vi "DAQ_pp3c_AudioLoadBuffersTasks.vi"(5 "Daq status in":T1={"Sound AO"="Dev6/ao0", "Shock intesity AO"="Dev6/ao1", "Code_LED DO"="Dev6/port1:2", "Switch DI"="Dev6/port1/line0", "Webcam"="cam9", "Sound AO task"="", "Sound card task"=0, "Shock intensity AO task"="", "Code_LED DO task"="", "Switch DI task"="", "AO <=> Sound card"=FALSE, "Sound card"=0, "sample rate"=100000.0, "Variable shock"=TRUE, "Webcam on"=FALSE, "Waveform memo"={"t0"=timestamp(0 s since 1904-01-01), "dt"=1.0, "Y"=[]}, "Tone trigger"="PFI1", "Master-9 DO"="PFI1", "Master-9 DO task"="Dev6/port0/line5:7", "Master-9 on"=TRUE} {"sample rate" min=8000.0; "Sound card task" format="%.0x"}, 7 "Waveform":waveform(dbl), 11 "error in (no error)":errorcluster) -> (6 "Daq status out":T1={"Sound AO"="Dev6/ao0", "Shock intesity AO"="Dev6/ao1", "Code_LED DO"="Dev6/port1:2", "Switch DI"="Dev6/port1/line0", "Webcam"="cam9", "Sound AO task"="", "Sound card task"=0, "Shock intensity AO task"="", "Code_LED DO task"="", "Switch DI task"="", "AO <=> Sound card"=FALSE, "Sound card"=0, "sample rate"=100000.0, "Variable shock"=TRUE, "Webcam on"=FALSE, "Waveform memo"={"t0"=timestamp(0 s since 1904-01-01), "dt"=1.0, "Y"=[]}, "Tone trigger"="PFI1", "Master-9 DO"="PFI1", "Master-9 DO task"="Dev6/port0/line5:7", "Master-9 on"=TRUE} {"sample rate" min=8000.0; "Sound card task" format="%.0x"}, 15 "error out":errorcluster)   [LabVIEW 2013]
uses:
  CTL_pp3c_DaqStatus.ctl
  <vilib>/userdefined/High Color/IMAQdx.ctl
  <vilib>/sound2/lvsound2.llb/Sound Output Task ID.ctl
  <vilib>/DAQmx/write.llb/DAQmx Write (Analog Wfm 1Chan NSamp).vi
  <vilib>/DAQmx/create/channels.llb/DAQmx Create Channel (AO-Voltage-Basic).vi
  <vilib>/DAQmx/configure/timing.llb/DAQmx Timing (Use Waveform).vi
  <vilib>/DAQmx/miscellaneous.llb/DAQmx Fill In Error Info.vi
  <resource>/objmgr/daqmx.rc
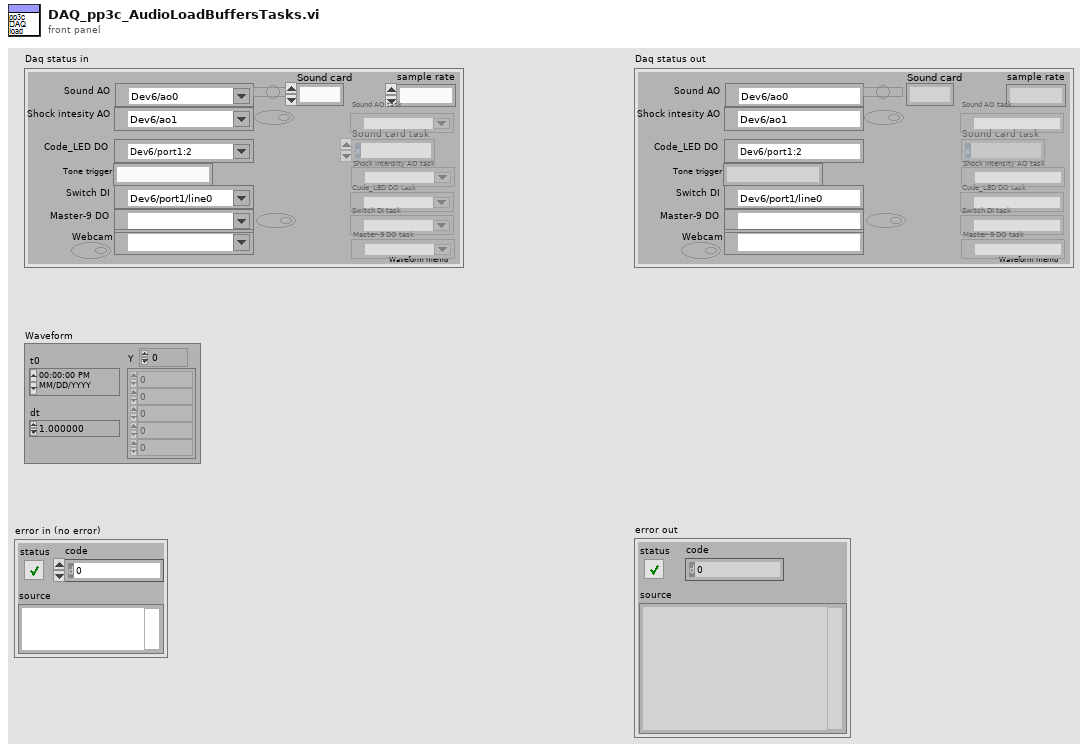
[diagram p1: front panel]
types:
  T1 = typedef "CTL_pp3c_DaqStatus.ctl" = cluster{"Sound AO":tag, "Shock intesity AO":tag, "Code_LED DO":tag, "Switch DI":tag, "Webcam":T2, "Sound AO task":refnum<k21>, "Sound card task":T3, "Shock intensity AO task":refnum<k21>, "Code_LED DO task":refnum<k21>, "Switch DI task":refnum<k21>, "AO <=> Sound card":bool, "Sound card":u32, "sample rate":dbl, "Variable shock":bool, "Webcam on":bool, "Waveform memo":waveform(dbl), "Tone trigger":string, "Master-9 DO":tag, "Master-9 DO task":refnum<k21>, "Master-9 on":bool}
  T2 = typedef "IMAQdx.ctl" = refnum<k21>
  T3 = typedef "Sound Output Task ID.ctl" = u32
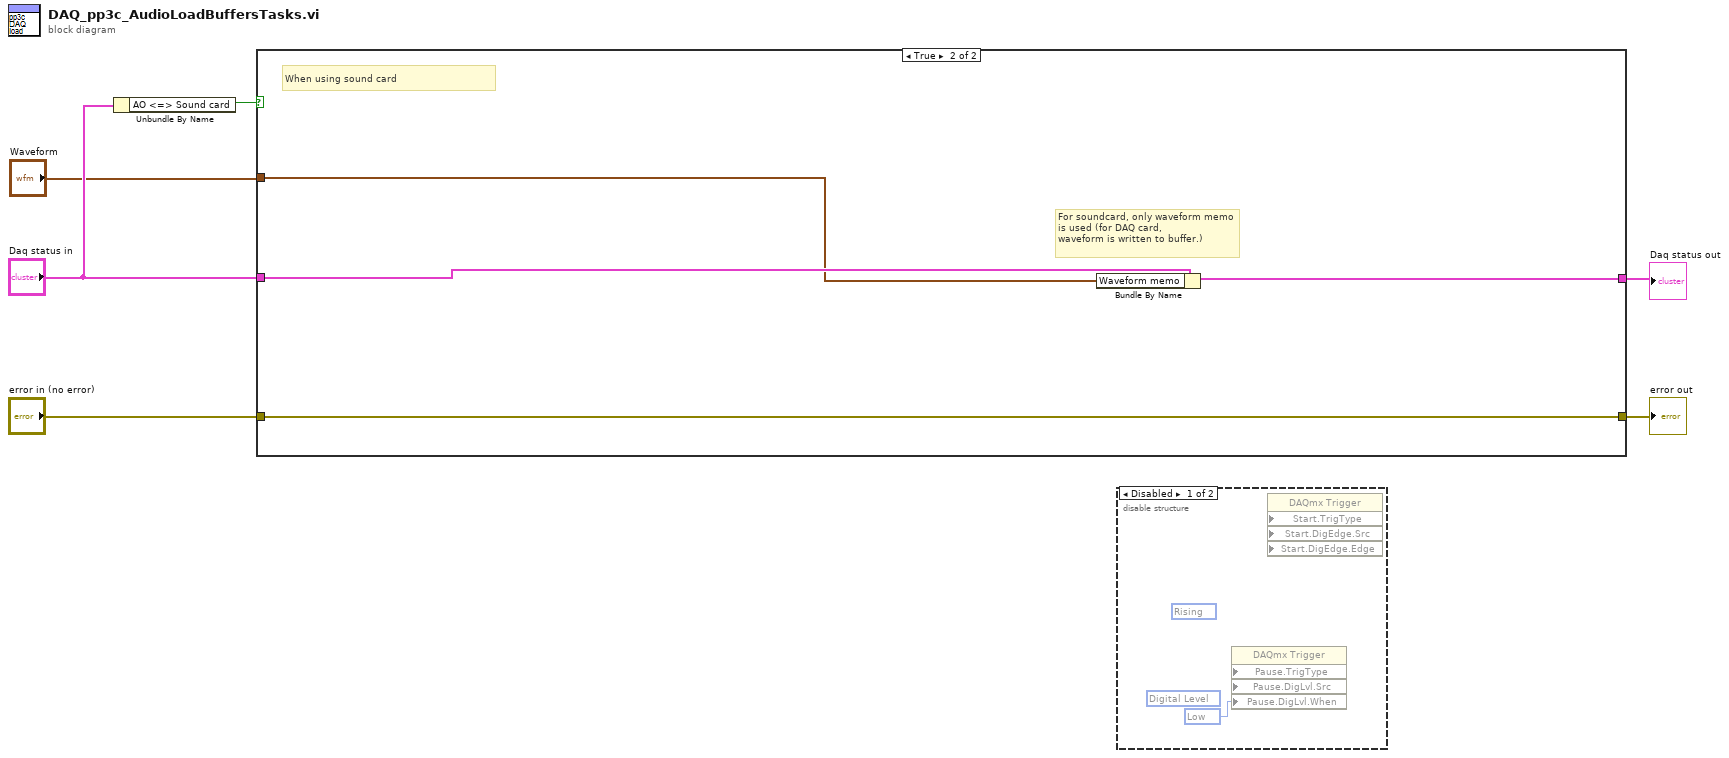
[diagram p0: block diagram]
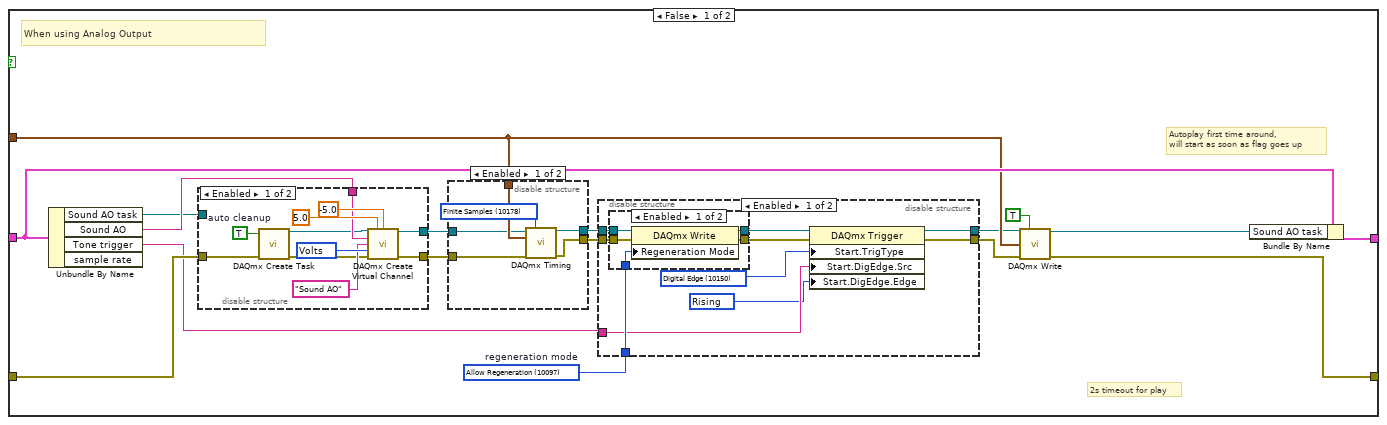
[diagram p3: hidden frame]
diagram:
  n1 = Unbundle By Name("Daq status in") -> ("AO <=> Sound card"=w6:bool)
  n2 = case shown="True" w6 {
    tunnel: "Daq status in" -> [w22 w66]
    tunnel: [w21 w67] -> w3
    tunnel: "error in (no error)" -> [w14 w64]
    tunnel: [w7 w64] -> w2
    tunnel: "Waveform" -> [w20 w65]
    frame False {
      w15 = 10097 items=["Allow Regeneration"=10097, "Do Not Allow Regeneration"=10158]  # regeneration mode
      # "2s timeout for play"
      # "Autoplay first time around,\nwill start as soon as flag goes up"
      # "When using Analog Output"
      n3 = Unbundle By Name(w22) -> ("Sound AO task"=w10:refnum<k21>, "Sound AO"=w17:tag, "Tone trigger"=w11:string)  [unwired: 1 out]
      n4 = disable-structure shown="Enabled" {
        disable-tunnel: [w38 w44] -> w19
        disable-tunnel: [w37 w43] -> w18
        disable-tunnel: w17 -> [w36 _]
        disable-tunnel: w14 -> [w33 w43]
        disable-tunnel: w10 -> [_ w44]
        frame Enabled {
          w35 = TRUE  # auto cleanup
          w42 = 10348 items=["Volts"=10348, "From Custom Scale"=10065] ("units")
          n5 = call <vilib>:"DAQmx Create Task.vi"("auto cleanup"=w35, "error in"=w33) -> ("task out"=w34:refnum<k21>, "error out"=w32:errorcluster)  [unwired: 12 in]
          n6 = call-poly <vilib>:"DAQmx Create Virtual Channel.vi"("task in"=w34, "maximum value"=5.0, "minimum value"=-5.0, "physical channels"=w36, "name to assign"="Sound AO", "units"=w42, "error in"=w32) -> ("task out"=w38:refnum<k21>, "error out"=w37:errorcluster)  [unwired: 7 in]
        }
        frame Disabled {
        }
      }
      n7 = disable-structure shown="Enabled" {
        disable-tunnel: w20 -> [w28 _]
        disable-tunnel: w19 -> [w27 w31]
        disable-tunnel: w18 -> [w26 w30]
        disable-tunnel: [w25 w30] -> w16
        disable-tunnel: [w24 w31] -> w9
        frame Enabled {
          w29 = 10178 items=["Finite Samples"=10178, "Continuous Samples"=10123, "Hardware Timed Single Point"=12522] ("sample mode")
          n8 = call-poly <vilib>:"DAQmx Timing.vi"("task/channels in"=w27, "sample mode"=w29, "waveform"=w28, "error in"=w26) -> ("task out"=w24:refnum<k21>, "error out"=w25:errorcluster)  [unwired: 10 in]
        }
        frame Disabled {
        }
      }
      n9 = disable-structure shown="Enabled" {
        disable-tunnel: w9 -> [w54 w63]
        disable-tunnel: w16 -> [w53 w62]
        disable-tunnel: w15 -> [w52 _]
        disable-tunnel: [w48 w63] -> w13
        disable-tunnel: [w47 w62] -> w12
        disable-tunnel: w11 -> [w49 _]
        frame Enabled {
          w46 = 10150 items=["Analog Edge"=10099, "Digital Edge"=10150, "Digital Pattern"=10398, "Analog Window"=10103, "None"=10230] ("Start.TrigType")
          w45 = 10280 items=["Rising"=10280, "Falling"=10171] ("Start.DigEdge.Edge")
          n10 = disable-structure shown="Enabled" {
            disable-tunnel: w54 -> [w59 w61]
            disable-tunnel: w53 -> [w58 w60]
            disable-tunnel: w52 -> [w57 _]
            disable-tunnel: [w56 w61] -> w51
            disable-tunnel: [w55 w60] -> w50
            frame Enabled {
              n11 = property class="DAQmx Write"(reference=w59, error in=w58, "Regeneration Mode"=w57) -> (reference out=w56:refnum<k21>, error out=w55:errorcluster)
            }
            frame Disabled {
            }
          }
          n12 = property class="DAQmx Trigger"(reference=w51, error in=w50, "Start.TrigType"=w46, "Start.DigEdge.Src"=w49, "Start.DigEdge.Edge"=w45) -> (reference out=w48:refnum<k21>, error out=w47:errorcluster)
        }
        frame Disabled {
        }
      }
      n13 = call-poly <vilib>:"DAQmx Write.vi"("task/channels in"=w13, "auto start"=TRUE, "data"=w20, "error in"=w12) -> ("task out"=w8:refnum<k21>, "error out"=w7:errorcluster)  [unwired: 9 in, 1 out]
      n14 = Bundle By Name(cluster=w22, "Sound AO task"=w8) -> (w21:T1)
    }
    frame True {
      # "When using sound card"
      # "For soundcard, only waveform memo is used (for DAQ card,\nwaveform is written to buffer.)"
      n15 = Bundle By Name(cluster=w66, "Waveform memo"=w65) -> (w67:T1)
    }
  }
  "Daq status out" <- w3
  "error out" <- w2
  n16 = disable-structure shown="Disabled" {
    frame Disabled {
      w68 = 10214 items=["High"=10192, "Low"=10214] ("Pause.DigLvl.When")
      (unwired) 10152 items=["Analog Level"=10101, "Analog Window"=10103, "Digital Level"=10152, "Digital Pattern"=10398, "None"=10230] ("Pause.TrigType")
      (unwired) 10280 items=["Rising"=10280, "Falling"=10171] ("Start.DigEdge.Edge")
      n17 = property class="DAQmx Trigger" props=["Pause.TrigType", "Pause.DigLvl.Src", "Pause.DigLvl.When"]("Pause.DigLvl.When"=w68) -> ()  [unwired: 4 in, 2 out]
      n18 = property class="DAQmx Trigger" props=["Start.TrigType", "Start.DigEdge.Src", "Start.DigEdge.Edge"]() -> ()  [unwired: 5 in, 2 out]
    }
    frame Enabled {
    }
  }
